vi "ControlPID_VI.vi"() -> ()   [LabVIEW 2026]
uses:
  <vilib>/Utility/miscctls.llb/LVPointTypeDef.ctl
  Control/Ctrl_ControlPIDEvent.ctl
  Control/Ctrl_QueuePID.ctl
  <vilib>/addons/control/pid/NI_PID_pid.lvlib
  GlobalVariable/Muestreo.vi
  Control/Ctrl_Articulacion_PIDGui.ctl
  <vilib>/addons/control/pid/pid.llb/PID (DBL).vi
  Control/Ctrl_EscrituraComandos.ctl
  Control/Cluster_ControlPID_Subpanel.ctl
panel:
  in  "Td":dbl
  in  "TI":dbl
  in  "Setpoint":i32
  in  "Articulacion":T1 caption="Articulación"
  out "PWM":i32
  out "Error Actual":i32
  in  "KP":dbl caption="Gauge"
  out "Chart":cluster{"Setpoint":i32, "Pasos":i32}(graph) caption="Waveform Chart - Dark"
  out "time string":string
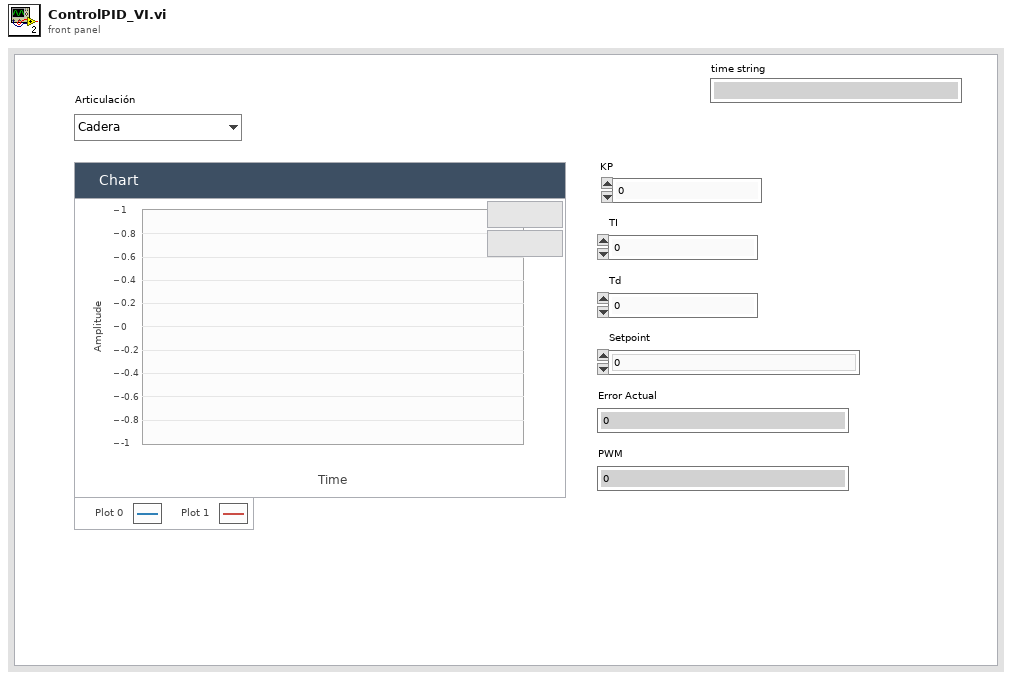
[diagram p1: front panel]
types:
  T1 = typedef "Ctrl_Articulacion_PIDGui.ctl" = enum16{"Cadera", "Hombro", "Codo", "Antebrazo", "Muñeca", "Gripper"}
  T2 = typedef "Ctrl_QueuePID.ctl" = enum16{"Start", "Stop", "Idle", "ObtainValues"}
  T3 = cluster{"Estado":T2, "Array_Pasos":i32[], "Articulacion ":T1}
  T4 = typedef "Ctrl_ControlPIDEvent.ctl" = enum16{"Set Ref", "Update Enc", "Stop", "Get Ref"}
  T5 = typedef "LVPointTypeDef.ctl" = cluster{"Horizontal":i16, "Vertical":i16}
  T6 = typedef "Cluster_ControlPID_Subpanel.ctl" = cluster{"Estado":T2, "Array_Pasos":i32[], "Articulacion ":T1}
  T7 = typedef "Ctrl_Array_Enc_Out.ctl" = T8[]
  T8 = typedef "Ctr_Enc_Values.ctl" = cluster{"Datos6_Motores":T9, "Errores":T11, "new_data?":bool}
  T9 = typedef "Ctrl_datos6motores_final.ctl" = cluster{"M_cadera":T10, "M_hombro":T10, "M_codo":T10, "M_antebrazo":T10, "M_muneca":T10, "M_gripper":T10}
  T10 = typedef "Ctrl_Motores_Valores.ctl" = cluster{"Pasos":i32, "Vueltas":i16, "Velocidad":dbl, "Reserva1":u8, "Reserva2":u8}
  T11 = typedef "Ctrl_Errores.ctl" = cluster{"Contador_correcto":u32, "Contador_errores":u32, "Edo_conex":u32}
  T12 = typedef "Ctrl_EscrituraComandos.ctl" = enum16{"SEND PID", "GET REF", "SEND MANUAL COM", "SEND ESP32", "SET REF"}
  T13 = cluster{"proportional gain (Kc)":dbl, "integral time (Ti, min)":dbl, "derivative time (Td, min)":dbl}
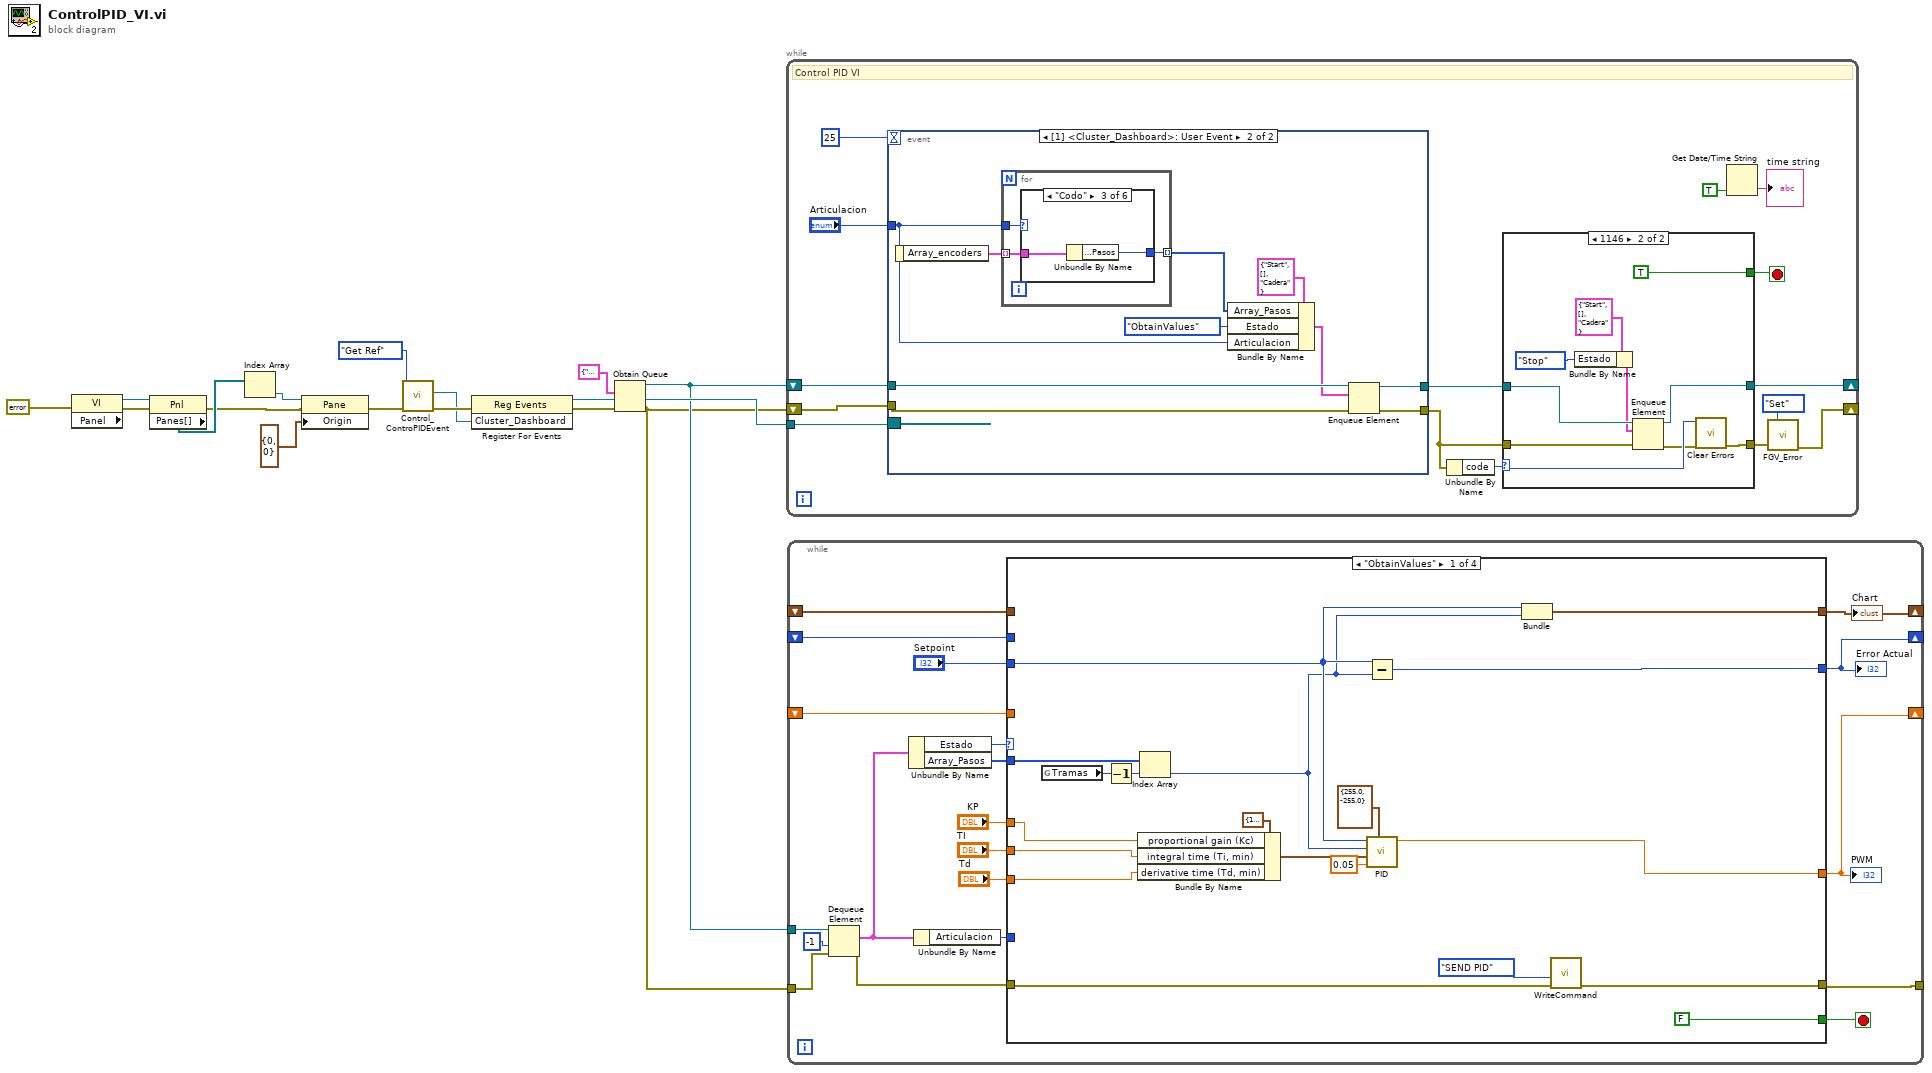
[diagram p0: block diagram]
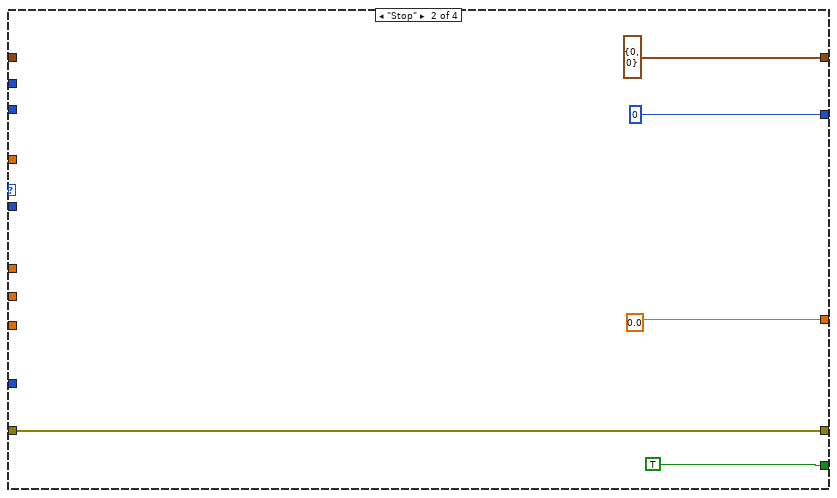
[diagram p2: hidden frame]
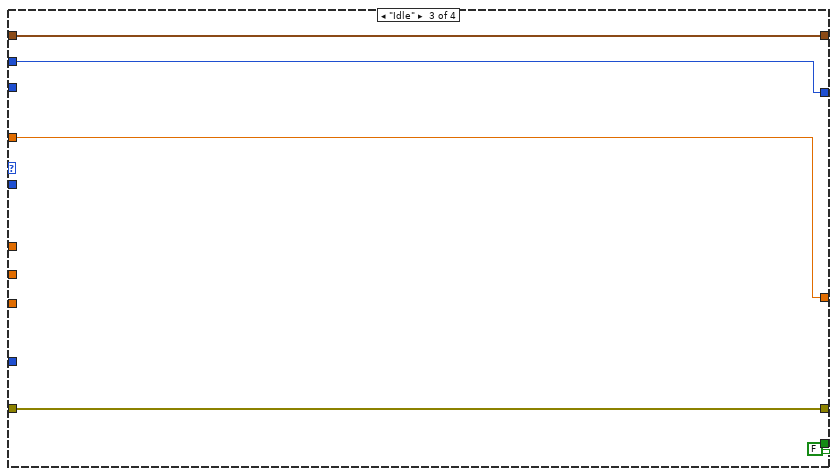
[diagram p3: hidden frame]
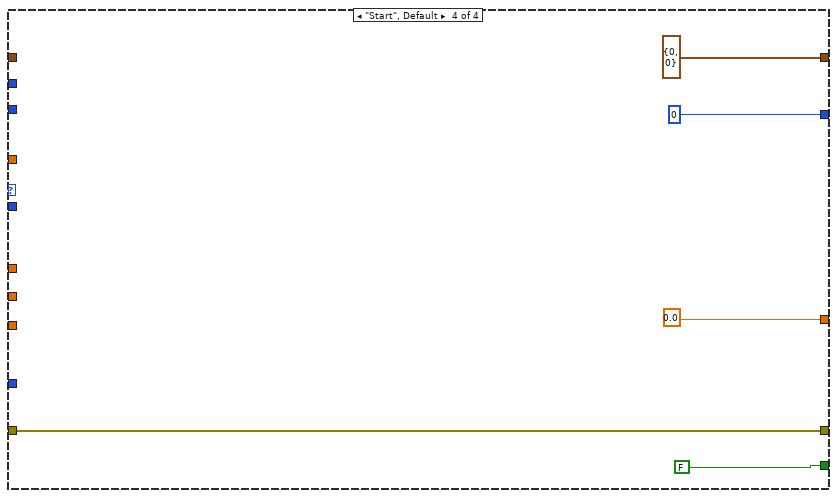
[diagram p4: hidden frame]
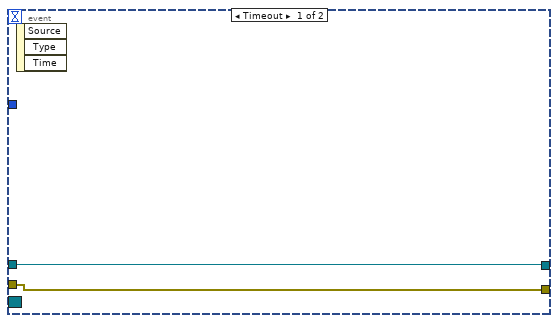
[diagram p5: hidden frame]
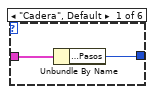
[diagram p6: hidden frame]
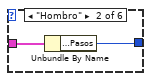
[diagram p7: hidden frame]
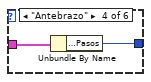
[diagram p8: hidden frame]
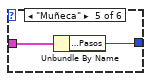
[diagram p9: hidden frame]
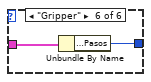
[diagram p10: hidden frame]
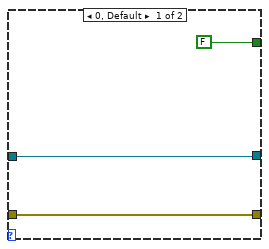
[diagram p11: hidden frame]
diagram:
  n1 = property class="VI"(error in=errorcluster {"status"=FALSE, "code"=0, "source"=""} ("error in (no error)")) -> (error out=w15:errorcluster, "Panel"=w16:refnum<vi>)  [unwired: 1 in, 1 out]
  n2 = property class="Pnl"(reference=w16, error in=w15) -> (error out=w12:errorcluster, "Panes[]"=w14:refnum<vi>[])  [unwired: 1 out]
  n3 = Index Array(array=w14) -> (element=w13:refnum<vi>)  [unwired: 1 in]
  n4 = property class="Pane"(reference=w13, error in=w12, "Origin"=T5 {"Horizontal"=0, "Vertical"=0}) -> (error out=w8:errorcluster)  [unwired: 1 out]
  n5 = call "Control_ControPIDEvent.vi"("error in"=w8, "Estado"=Ctrl_ControlPIDEvent."Get Ref") -> ("error out"=w7:errorcluster, "Cluster_Dashboard"=w6:refnum<user-event>)  [unwired: 8 in]
  n6 = register-events(error in=w7, w6) -> (reference out=w5:refnum<event-registration>, error out=w4:errorcluster)  [unwired: 1 in]
  n7 = Obtain Queue(element data type=T3 {"Estado"=enum."Start", "Array_Pasos"=[], "Articulacion "=enum."Cadera"}, error in (no error)=w4) -> (queue out=w3:refnum<queue>, error out=w2:errorcluster)  [unwired: 3 in, 1 out]
  n8 = while {
    shift-right: [w29] -> _
    shift-left: w2 -> [w25]
    tunnel: w5 -> [w24]
    shift-right: [w17] -> _
    shift-left: w3 -> [w19]
    stop <- w31 stop-if-true
    # "Control PID VI"
    n9 = event shown="[1] <Cluster_Dashboard>: User Event" {
      selector: w24 -> [_ _]
      dyn-events: _ -> [_ _]
      timeout: 25 -> [_ _]
      tunnel: w25 -> [w33 w41]
      tunnel: [w33 w42] -> w22
      tunnel: "Articulacion" -> [_ w35]
      tunnel: w19 -> [w32 w40]
      tunnel: [w32 w36] -> w18
      event Timeout {
        n10 = event-data() -> ()  [unwired: 1 in, 3 out]
      }
      event User Event {
        n11 = event-data() -> ("Array_encoders"=w43:T7)  [unwired: 1 in]
        n12 = for {
          tunnel: w43 -> [w46] mode=indexing
          tunnel: w35 -> [w45]
          tunnel: [w44] -> w38 mode=indexing
          n13 = case shown="\"Codo\"" w45 {
            tunnel: w46 -> [w48 w50 w52 w54 w56 w58]
            tunnel: [w47 w49 w51 w53 w55 w57] -> w44
            frame "Cadera", Default {
              n14 = Unbundle By Name(w48) -> ("Datos6_Motores.M_cadera.Pasos"=w47:i32)
            }
            frame "Hombro" {
              n15 = Unbundle By Name(w50) -> ("Datos6_Motores.M_hombro.Pasos"=w49:i32)
            }
            frame "Codo" {
              n16 = Unbundle By Name(w52) -> ("Datos6_Motores.M_codo.Pasos"=w51:i32)
            }
            frame "Antebrazo" {
              n17 = Unbundle By Name(w54) -> ("Datos6_Motores.M_antebrazo.Pasos"=w53:i32)
            }
            frame "Muñeca" {
              n18 = Unbundle By Name(w56) -> ("Datos6_Motores.M_muneca.Pasos"=w55:i32)
            }
            frame "Gripper" {
              n19 = Unbundle By Name(w58) -> ("Datos6_Motores.M_gripper.Pasos"=w57:i32)
            }
          }
        }
        n20 = Bundle By Name(cluster=T6 {"Estado"=enum."Start", "Array_Pasos"=[], "Articulacion "=enum."Cadera"}, "Array_Pasos"=w38, "Estado"=Ctrl_QueuePID."ObtainValues", "Articulacion"=w35) -> (w34:T6)
        n21 = Enqueue Element(queue=w40, element=w34, error in (no error)=w41) -> (queue out=w36:refnum<queue>, error out=w42:errorcluster)  [unwired: 1 in, 1 out]
      }
    }
    n22 = Unbundle By Name(w22) -> ("code"=w21:i32)
    n23 = case shown="1146" w21 {
      selector: w21 -> [_ w71]
      tunnel: [FALSE TRUE] -> w31
      tunnel: w22 -> [w60 w68]
      tunnel: [w60 w69] -> w30
      tunnel: w18 -> [w59 w66]
      tunnel: [w59 w65] -> w17
      frame 0, Default {
      }
      frame 1146 {
        n24 = Bundle By Name(cluster=T6 {"Estado"=enum."Start", "Array_Pasos"=[], "Articulacion "=enum."Cadera"}, "Estado"=Ctrl_QueuePID."Stop") -> (w63:T6)
        n25 = Enqueue Element(queue=w66, element=w63, error in (no error)=w68) -> (queue out=w65:refnum<queue>, error out=w67:errorcluster)  [unwired: 1 in, 1 out]
        n26 = call <vilib>:"Clear Errors.vi"("error in (no error)"=w67, "specific error code to clear (0: all)"=w71) -> ("error out"=w69:errorcluster)  [unwired: 4 in, 1 out]
      }
    }
    n27 = Get Date/Time String(want seconds? (F)=TRUE) -> (time string=→"time string":string)  [unwired: 2 in, 1 out]
    n28 = call "FGV_Error.vi"("error_in_loop"=w30, "Estado"=enum16{"Set", "Get"}."Set") -> ("error out"=w29:errorcluster)  [unwired: 9 in]
  }
  n29 = while {
    shift-right: [w79] -> _
    shift-left: _ -> [w77]
    shift-right: [w80] -> _
    shift-left: _ -> [w78]
    tunnel: w3 -> [w89]
    tunnel: w2 -> [w91]
    tunnel: [w76] -> _
    shift-right: [w75] -> _
    shift-left: _ -> [w74]
    stop <- w81 stop-if-true
    n30 = Dequeue Element(queue=w89, timeout in ms (-1)=-1, error in (no error)=w91) -> (element=w73:T3, error out=w90:errorcluster)  [unwired: 2 out]
    n31 = Unbundle By Name(w73) -> ("Estado"=w88:T2, "Array_Pasos"=w86:i32[])
    n32 = Unbundle By Name(w73) -> ("Articulacion"=w72:T1)
    n33 = case shown="\"ObtainValues\"" w88 {
      tunnel: w90 -> [w93 w111 w116 w121]
      tunnel: w86 -> [w106 _ _ _]
      tunnel: "Setpoint" -> [w97 _ _ _]
      tunnel: "KP" -> [w102 _ _ _]
      tunnel: "TI" -> [w101 _ _ _]
      tunnel: "Td" -> [w100 _ _ _]
      tunnel: [FALSE TRUE FALSE FALSE] -> w81
      tunnel: [w99 0.0 ("output") w119 0.0 ("output")] -> w79
      tunnel: [w98 0 w118 0] -> w80
      tunnel: w78 -> [_ _ w118 _]
      tunnel: w77 -> [_ _ w119 _]
      tunnel: [w94 w111 w116 w121] -> w76
      tunnel: [w95 cluster{"Setpoint":i32, "Pasos":i32} {"Setpoint"=0, "Pasos"=0} w117 cluster{"Setpoint":i32, "Pasos":i32} {"Setpoint"=0, "Pasos"=0}] -> w75
      tunnel: w74 -> [_ _ w117 _]
      tunnel: w72 -> [_ _ _ _]
      frame "ObtainValues" {
        n34 = global read "Muestreo.vi" "Tramas"() -> (w104:i32)
        n35 = Decrement(x=w104) -> (x-1=w105:i32)
        n36 = Bundle By Name(cluster=T13 {"proportional gain (Kc)"=1.0, "integral time (Ti, min)"=0.01, "derivative time (Td, min)"=0.0} ("PID gains"), "proportional gain (Kc)"=w102, "integral time (Ti, min)"=w101, "derivative time (Td, min)"=w100) -> (w108:T13)
        n37 = Index Array(array=w106, index=w105) -> (element=w96:i32)
        n38 = Subtract(x=w97, y=w96) -> (x-y=w98:i32)
        n39 = call-poly <vilib>:"PID.vi"("output range"=cluster{"output high":dbl, "output low":dbl} {"output high"=255.0, "output low"=-255.0}, "dt (s)"=0.05, "PID gains"=w108, "process variable"=w96, "setpoint"=w97) -> ("output"=w99:dbl)  [unwired: 5 in, 1 out]
        n40 = Bundle("Setpoint"=w97, "Pasos"=w96) -> (w95:cluster{"Setpoint":i32, "Pasos":i32})  [unwired: 1 in]
        n41 = call "WriteCommand.vi"("error in"=w93, "Com_Escribir"=Ctrl_EscrituraComandos."SEND PID") -> ("error out"=w94:errorcluster)  [unwired: 8 in, 1 out]
      }
      frame "Stop" {
      }
      frame "Idle" {
      }
      frame "Start", Default {
      }
    }
    "Error Actual" <- w80
    "PWM" <- w79
    "Chart" <- w75
  }
